vi "Maquina_D_Eventos.vi"() -> ()   [LabVIEW 2021]
uses:
  Control 1.ctl
panel:
  in  "Stop Button":bool
  out "Motor Derecha":bool
  out "Motor Izquierda":bool
  in  "Sensor":bool
  # "Mendoza Meza Manuel Everardo"
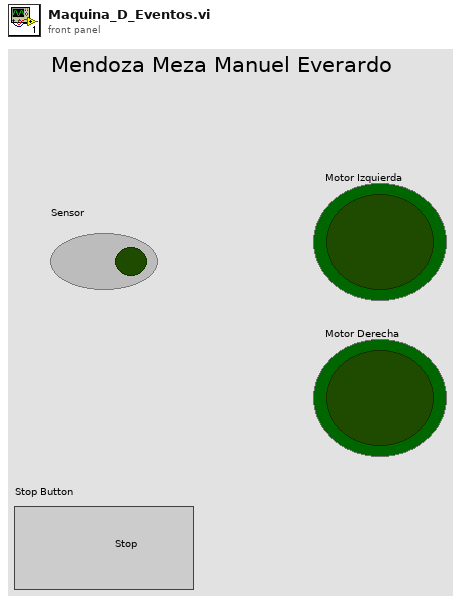
[diagram p1: front panel]
types:
  T1 = typedef "Control 1.ctl" = enum16{"Inicializacion", "Espera", "Giro1", "Giro2", "Detener"}
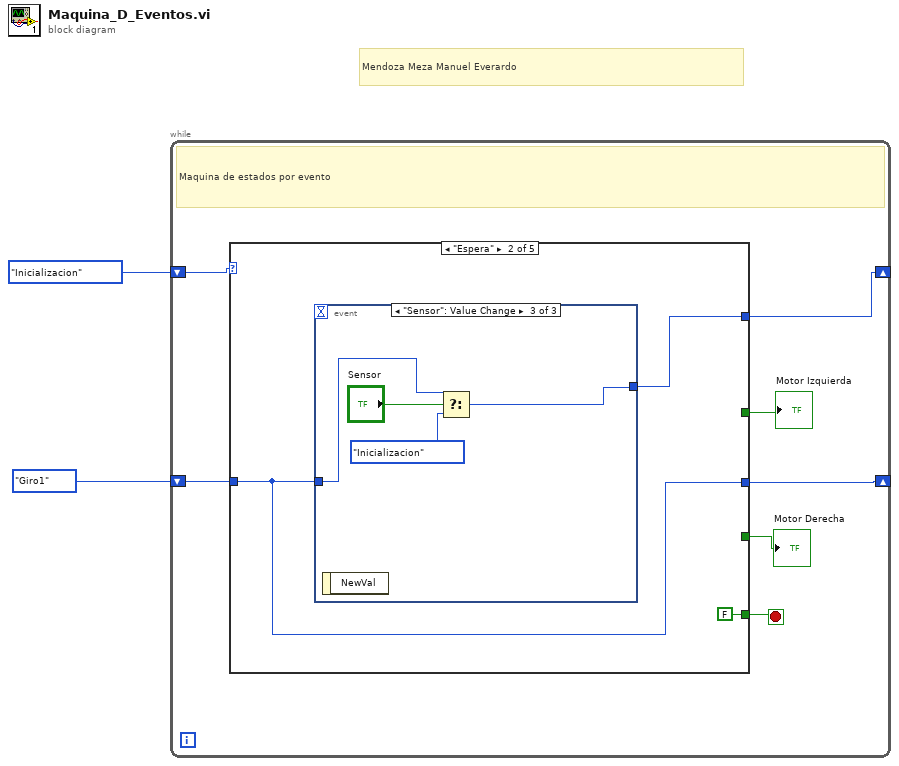
[diagram p0: block diagram]
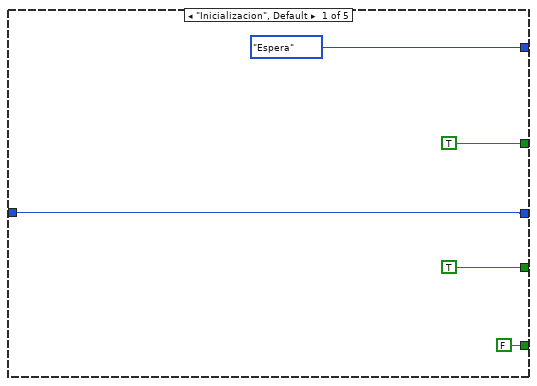
[diagram p2: hidden frame]
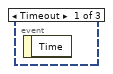
[diagram p3: hidden frame]
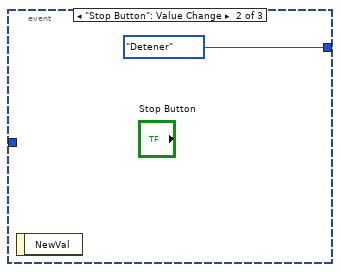
[diagram p4: hidden frame]
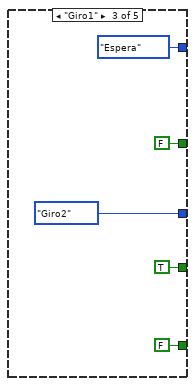
[diagram p5: hidden frame]
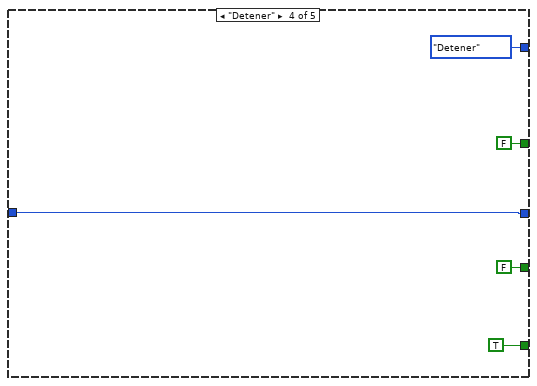
[diagram p6: hidden frame]
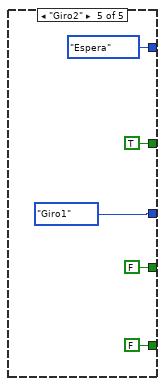
[diagram p7: hidden frame]
diagram:
  # "Mendoza Meza Manuel Everardo"
  n1 = while {
    shift-right: [w6] -> _
    shift-left: Control_1."Inicializacion" -> [w9]
    shift-right: [w3] -> _
    shift-left: Control_1."Giro1" -> [w4]
    stop <- w5 stop-if-true
    # "Maquina de estados por evento"
    n2 = case shown="\"Espera\"" w9 {
      tunnel: [TRUE _ FALSE FALSE TRUE] -> w8
      tunnel: [TRUE _ TRUE FALSE FALSE] -> w7
      tunnel: [Control_1."Espera" w16 Control_1."Espera" Control_1."Detener" Control_1."Espera"] -> w6
      tunnel: [FALSE FALSE FALSE TRUE FALSE] -> w5
      tunnel: w4 -> [w10 w15 _ w28 _]
      tunnel: [w10 w15 Control_1."Giro2" w28 Control_1."Giro1"] -> w3
      frame "Inicializacion", Default {
      }
      frame "Espera" {
        n3 = event shown="[2] \"Sensor\": Value Change" {
          selector: _ -> [_ _ _]
          dyn-events: _ -> [_ _ _]
          timeout: _ -> [_ _ _]
          tunnel: [_ Control_1."Detener" w19] -> w16
          tunnel: w15 -> [_ _ w21]
          event Timeout {
            n4 = event-data() -> ()  [unwired: 1 in, 1 out]
          }
          event "Stop Button": Value Change {
            n5 = event-data() -> ()  [unwired: 1 in, 1 out]
          }
          event "Sensor": Value Change {
            n6 = event-data() -> ()  [unwired: 1 in, 1 out]
            n7 = Select(t=w21, s="Sensor", f=Control_1."Inicializacion") -> (s? t:f=w19:T1)
          }
        }
      }
      frame "Giro1" {
      }
      frame "Detener" {
      }
      frame "Giro2" {
      }
    }
    "Motor Izquierda" <- w8
    "Motor Derecha" <- w7
  }
